vi "SEQ FGV.vi"(7 "Enum":enum16{"Read", "Write"}(ring), 8 "error in (no error)":errorcluster, 11 "Seq data in":T1 {"Launch Time" format="%<%x %.3X>T"}) -> (0 "error out":errorcluster, 3 "Seq data out":T1)   [LabVIEW 2022 SP3]
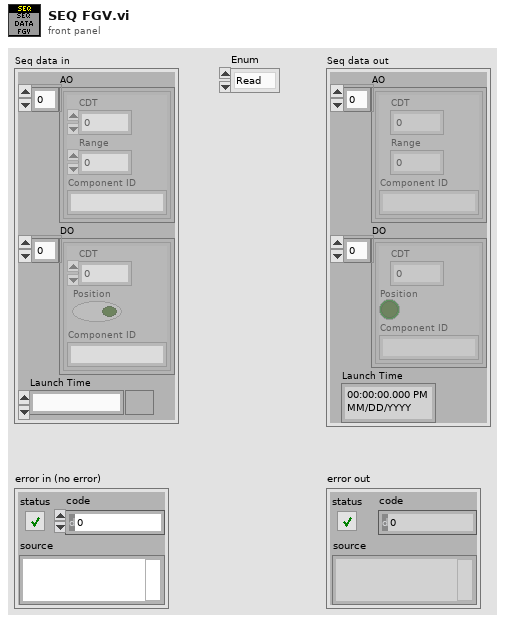
[diagram p1: front panel]
types:
  T1 = cluster{"AO":cluster{"CDT":dbl, "Range":dbl, "Component ID":string}[], "DO":cluster{"CDT":dbl, "Position":bool, "Component ID":string}[], "Launch Time":timestamp}
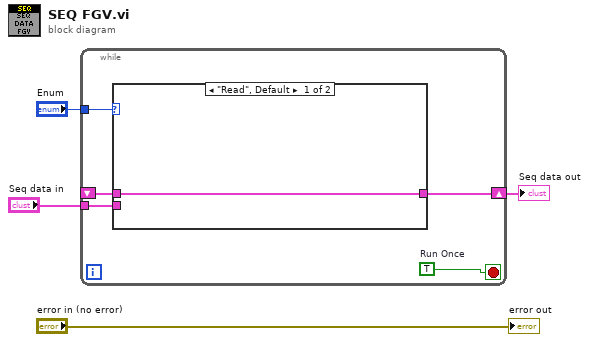
[diagram p0: block diagram]
diagram:
  n1 = while {
    shift-right: [w5] -> w1
    shift-left: _ -> [w8]
    tunnel: "Enum" -> [w7]
    tunnel: "Seq data in" -> [w6]
    stop <- w9 stop-if-true
    w9 = TRUE  # Run Once
    n2 = case shown="\"Read\", Default" w7 {
      tunnel: w8 -> [w10 _]
      tunnel: w6 -> [_ w11]
      tunnel: [w10 w11] -> w5
      frame "Read", Default {
      }
      frame "Write" {
      }
    }
  }
  "Seq data out" <- w1
  "error out" <- "error in (no error)"
